vi "dfd_Validate Input Dynamic Range.vi"(8 "error in (no error)":errorcluster, 10 "input range":dbl=10.0) -> (0 "error out":errorcluster)   [LabVIEW 2017, in "NI_DigFilter_FXP.lvlib"]
uses:
  <vilib>/addons/Digital Filter Design/NI_DigFilter_FXP.lvlib
  <vilib>/addons/Digital Filter Design/_Misc.llb/dfd_Error Handlers (Single).vi
  <vilib>/addons/Digital Filter Design/NI_DigFilterLicensed.lvlib
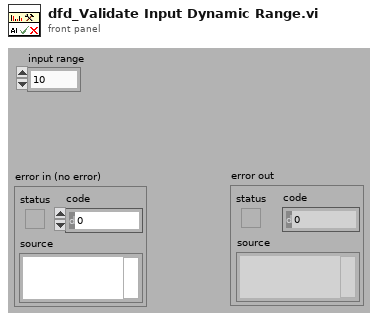
[diagram p1: front panel]
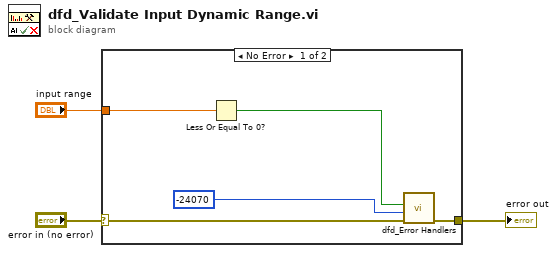
[diagram p0: block diagram]
diagram:
  n1 = case shown="No Error" "error in (no error)" {
    selector: "error in (no error)" -> [w8 w9]
    tunnel: [w7 w9] -> w2
    tunnel: "input range" -> [w5 _]
    frame No Error {
      n2 = Less Or Equal To 0?(x=w5) -> (x <= 0?=w4:bool)
      n3 = call-poly <vilib>:"dfd_Error Handlers.vi"("error in (no error)"=w8, "error code"=-24070 ("ERR_INVALID_INPUT_RANGE"), "condition failed?"=w4) -> ("error out"=w7:errorcluster)  [unwired: 8 out]
    }
    frame Error {
    }
  }
  "error out" <- w2
